vi "Menu-Start Imp.vi"(8 "error in":errorcluster, 11 "Menu in":refnum<k9>) -> ()   [LabVIEW 2016, in "CML UI.lvlib"]
uses:
  CML UI.lvlib
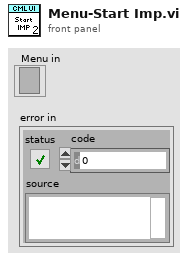
[diagram p1: front panel]
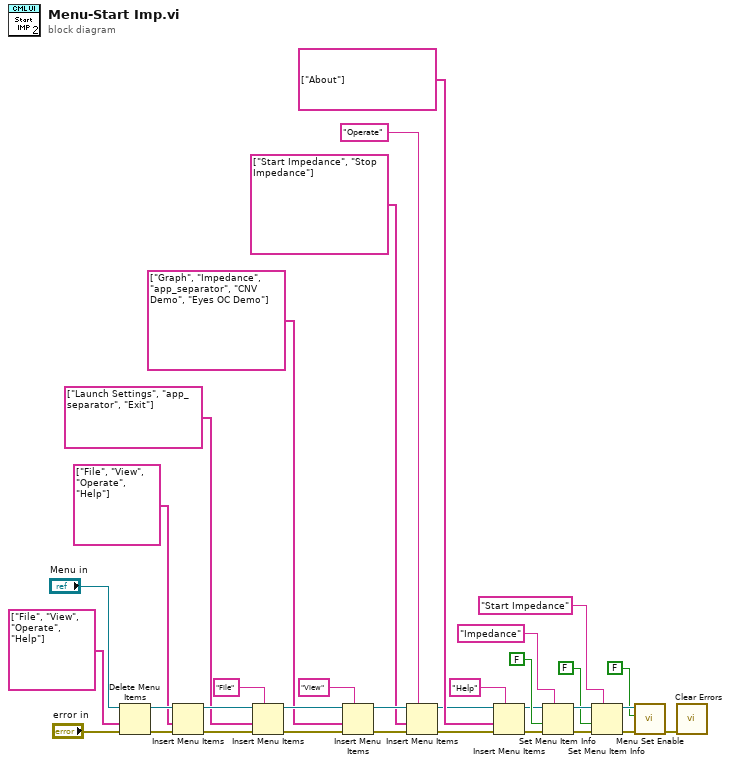
[diagram p0: block diagram]
diagram:
  n1 = Delete Menu Items(6:"error in", 7:string[] ["File", "View", "Operate", "Help"] ("L10n_item tags 1"), 9:"Menu in") -> (0:w34:errorcluster, 3:w33:refnum<k9>)  [unwired: 1 in]
  n2 = Insert Menu Items(6:w34, 7:string[] ["File", "View", "Operate", "Help"] ("L10n_item tags 1"), 9:w33) -> (0:w18:errorcluster, 3:w20:refnum<k9>)  [unwired: 3 in, 1 out]
  n3 = Insert Menu Items(5:"File" ("L10n_menu tag"), 6:w18, 7:string[] ["Launch Settings", "app_separator", "Exit"] ("L10n_item tags 2"), 9:w20) -> (0:w13:errorcluster, 3:w14:refnum<k9>)  [unwired: 2 in, 1 out]
  n4 = Insert Menu Items(5:"View" ("L10n_menu tag"), 6:w13, 7:string[] ["Graph", "Impedance", "app_separator", "CNV Demo", "Eyes OC Demo"] ("L10n_item tags 2"), 9:w14) -> (0:w9:errorcluster, 3:w10:refnum<k9>)  [unwired: 2 in, 1 out]
  n5 = Insert Menu Items(5:"Operate" ("L10n_menu tag"), 6:w9, 7:string[] ["Start Impedance", "Stop Impedance"] ("L10n_item tags 2"), 9:w10) -> (0:w23:errorcluster, 3:w22:refnum<k9>)  [unwired: 2 in, 1 out]
  n6 = Insert Menu Items(5:"Help" ("L10n_menu tag"), 6:w23, 7:string[] ["About"] ("L10n_item tags 2"), 9:w22) -> (0:w27:errorcluster, 3:w25:refnum<k9>)  [unwired: 2 in, 1 out]
  n7 = Set Menu Item Info(7:"Impedance" ("item tag"), 8:w27, 9:FALSE ("enabled"), 11:w25) -> (0:w32:errorcluster, 3:w31:refnum<k9>)  [unwired: 3 in]
  n8 = Set Menu Item Info(7:"Start Impedance" ("item tag"), 8:w32, 9:FALSE ("enabled"), 11:w31) -> (0:w4:errorcluster, 3:w3:refnum<k9>)  [unwired: 3 in]
  n9 = call "Menu Set Enable.vi"("error in (no error)"=w4, "enabled ?"=FALSE, "Menu in"=w3) -> ("error out"=w2:errorcluster)  [unwired: 7 in, 1 out]
  n10 = call <vilib>:"Clear Errors.vi"("error in (no error)"=w2) -> ()  [unwired: 5 in, 2 out]
